vi "D_2Darray_to_pict.vi"(8 "error in (no error)":errorcluster, 11 "2D array in":u8[][](array[numeric])) -> (0 "error out":errorcluster, 3 "gray scale picture out":picture)   [LabVIEW 2016]
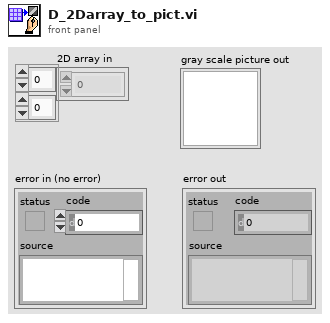
[diagram p1: front panel]
types:
  T1 = typedef "imagedata.ctl" = cluster{"image type":i32, "image depth":i32, "image":u8[], "mask":u8[], "colors":u32[], "Rectangle":cluster{"left":i16, "top":i16, "right":i16, "bottom":i16}}
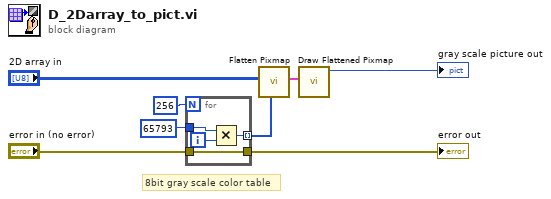
[diagram p0: block diagram]
diagram:
  # "8bit gray scale color table"
  n1 = for {
    N: 256 -> [_]
    tunnel: 65793 -> [w11]
    tunnel: [w10] -> w7 mode=indexing
    tunnel: "error in (no error)" -> [w9]
    tunnel: [w9] -> w1
    i -> [w12]
    n2 = Multiply(x=w11, y=w12) -> (x*y=w10:i32)
  }
  "error out" <- w1
  n3 = call <vilib>:"Flatten Pixmap.vi"("colors"=w7, "8-bit pixmap"="2D array in") -> ("image data"=w5:T1)  [unwired: 9 in]
  n4 = call <vilib>:"Draw Flattened Pixmap.vi"("image data"=w5) -> ("new picture"=→"gray scale picture out":picture)  [unwired: 8 in]
